vi "dht11_VisaSerial.vi"() -> ()   [LabVIEW 2021]
uses:
  <vilib>/Instr/_visa.llb/VISA Configure Serial Port (Instr).vi
panel:
  in  "Boolean":bool
  out "TEMPERATURA °C":dbl(slide) scale=0.0..50.0
  out "temperatura C":dbl
  in  "Cancel Button":bool
  out "read buffer":string
  in  "VISA resource name":refnum<visa-resource-name>
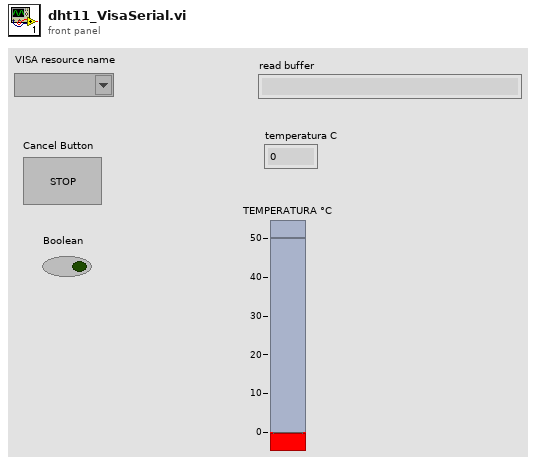
[diagram p1: front panel]
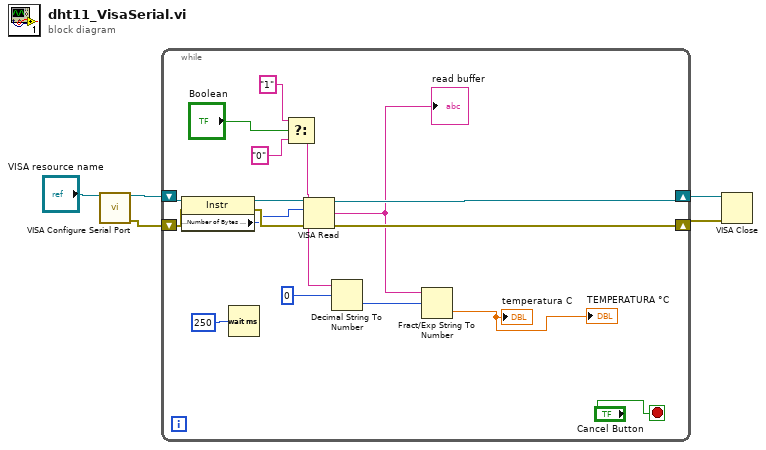
[diagram p0: block diagram]
diagram:
  n1 = call-poly "VISA Configure Serial Port"("VISA resource name"="VISA resource name") -> ("VISA resource name out"=w3:refnum<visa-resource-name>, "error out"=w4:errorcluster)  [unwired: 13 in]
  n2 = while {
    shift-right: [w13] -> w1
    shift-left: w4 -> [w22]
    shift-right: [w14] -> w2
    shift-left: w3 -> [w21]
    stop <- "Cancel Button" stop-if-true
    n3 = property class="Instr"(reference=w21, error in=w22) -> (reference out=w20:refnum<visa-resource-name>, error out=w19:errorcluster, "Serial Settings:Number of Bytes at Serial Port"=w18:u32)
    n4 = Wait (ms)(milliseconds to wait=u32 250) -> ()  [unwired: 1 out]
    n5 = Select(t="1", s="Boolean", f="0") -> (s? t:f=w9:string)
    n6 = VISA Read(VISA resource name=w20, byte count=w18, error in (no error)=w19) -> (VISA resource name out=w14:refnum<visa-resource-name>, read buffer=w7:string, error out=w13:errorcluster)  [unwired: 1 out]
    "read buffer" <- w7
    n7 = Decimal String To Number(string=w9, offset=0) -> (number=w8:i32)  [unwired: 1 in, 1 out]
    n8 = Fract/Exp String To Number(string=w7, offset=w8) -> (number=→"temperatura C" →"TEMPERATURA °C":dbl)  [unwired: 2 in, 1 out]
  }
  n9 = VISA Close(VISA resource name=w2, error in (no error)=w1) -> ()  [unwired: 1 out]
